vi "zad73.vi"() -> ()   [LabVIEW 2018]
uses:
  zad3states.ctl
panel:
  out "?":dbl(slide) scale=0.0..500.0
  in  "Draught Level":dbl(slide) scale=1.0..50.0
  in  "?":bool
  in  "?":bool
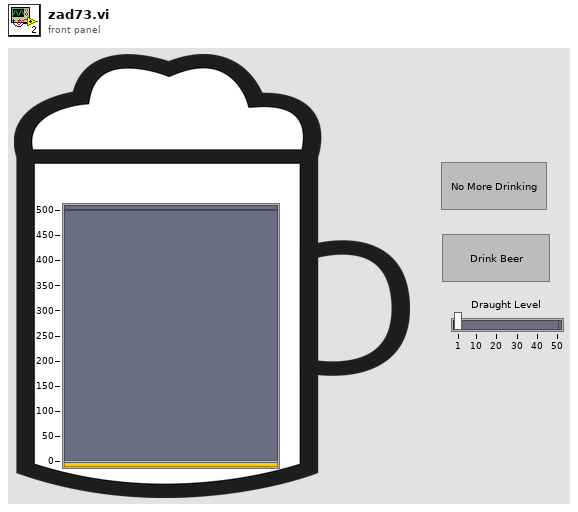
[diagram p1: front panel]
types:
  T1 = typedef "zad3states.ctl" = enum16{"Initialize", "Idle", "Drink", "Refill", "No more drinking", "End"}
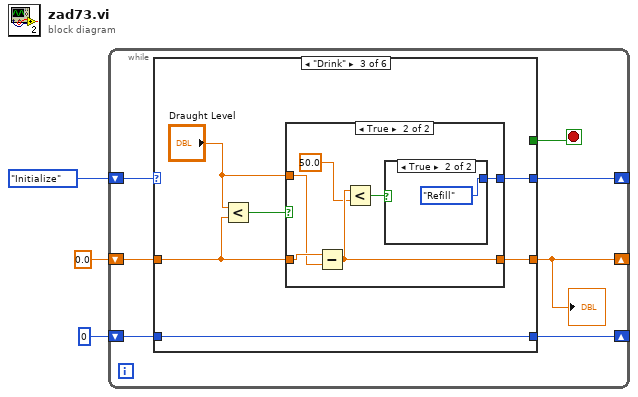
[diagram p0: block diagram]
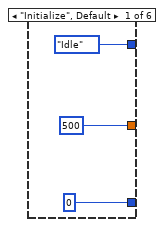
[diagram p2: hidden frame]
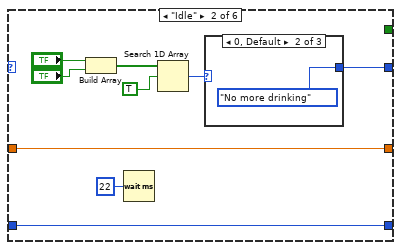
[diagram p3: hidden frame]
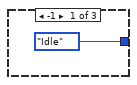
[diagram p4: hidden frame]
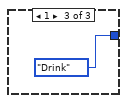
[diagram p5: hidden frame]
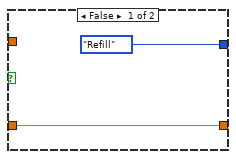
[diagram p6: hidden frame]
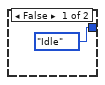
[diagram p7: hidden frame]
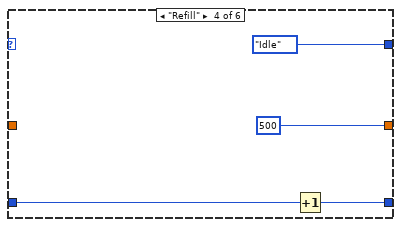
[diagram p8: hidden frame]
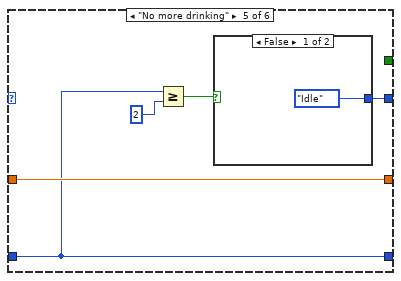
[diagram p9: hidden frame]
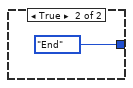
[diagram p10: hidden frame]
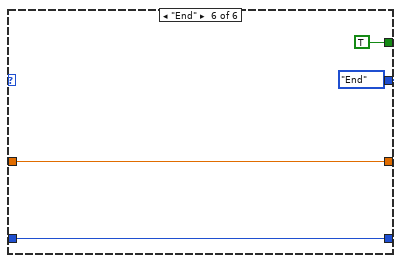
[diagram p11: hidden frame]
diagram:
  n1 = while {
    shift-right: [w9] -> _
    shift-left: zad3states."Initialize" -> [w10]
    shift-right: [w5] -> _
    shift-left: 0.0 -> [w6]
    shift-right: [w8] -> _
    shift-left: 0 -> [w7]
    stop <- w4 stop-if-true
    n2 = case shown="\"Drink\"" w10 {
      tunnel: [zad3states."Idle" w15 w30 zad3states."Idle" w46 zad3states."End"] -> w9
      tunnel: [500 w17 w28 500 w50 w55] -> w5
      tunnel: [0 w18 w27 w45 w49 w54] -> w8
      tunnel: w7 -> [_ w18 w27 w44 w49 w54]
      tunnel: w6 -> [_ w17 w29 _ w50 w55]
      tunnel: [_ _ _ _ _ TRUE] -> w4
      frame "Initialize", Default {
      }
      frame "Idle" {
        n3 = Build Array("?", "?") -> (w20:bool[])
        n4 = Wait (ms)(milliseconds to wait=u32 22) -> ()  [unwired: 1 out]
        n5 = Search 1D Array(1D array=w20, element=TRUE) -> (index of element=w16:i32)  [unwired: 1 in]
        n6 = case shown="0, Default" w16 {
          tunnel: [zad3states."Idle" zad3states."No more drinking" zad3states."Drink"] -> w15
          frame -1 {
          }
          frame 0, Default {
          }
          frame 1 {
          }
        }
      }
      frame "Drink" {
        n7 = Less?(x="Draught Level", y=w29) -> (x < y?=w31:bool)
        n8 = case shown="True" w31 {
          tunnel: [zad3states."Refill" w34] -> w30
          tunnel: w29 -> [w32 w39]
          tunnel: "Draught Level" -> [_ w38]
          tunnel: [w32 w36] -> w28
          frame False {
          }
          frame True {
            n9 = Subtract(x=w39, y=w38) -> (x-y=w36:dbl)
            n10 = Less?(x=w36, y=50.0) -> (x < y?=w37:bool)
            n11 = case shown="True" w37 {
              tunnel: [zad3states."Idle" zad3states."Refill"] -> w34
              frame False {
              }
              frame True {
              }
            }
          }
        }
      }
      frame "Refill" {
        n12 = Increment(x=w44) -> (x+1=w45:i32)
      }
      frame "No more drinking" {
        n13 = Greater Or Equal?(x=w49, y=2) -> (x >= y?=w47:bool)
        n14 = case shown="False" w47 {
          tunnel: [zad3states."Idle" zad3states."End"] -> w46
          frame False {
          }
          frame True {
          }
        }
      }
      frame "End" {
      }
    }
    "?" <- w5
  }
